vi "Handle_CMD_OFF.vi"(0 "reference in":refnum<class "Stand.lvclass">, 5 "error in (no error)":errorcluster) -> (14 "reference out":refnum<class "Stand.lvclass">, 19 "error out":errorcluster)   [LabVIEW 2019]
uses:
  Stand.lvclass
  D:/H4000/src/Device_class/Device.lvclass
  D:/H4000/src/Proccess_class/Proccess.lvclass
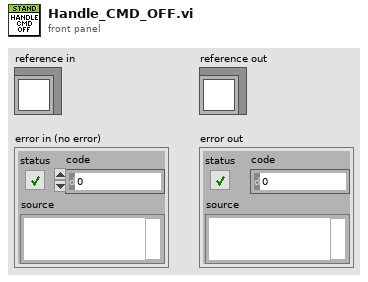
[diagram p1: front panel]
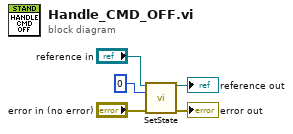
[diagram p0: block diagram]
diagram:
  n1 = call "SetState.vi"("reference in"="reference in", "State"=u16 0, "error in (no error)"="error in (no error)") -> ("reference out"=→"reference out":refnum<class "Stand.lvclass">, "error out"=→"error out":errorcluster)  [unwired: 11 in]
